vi "PulseTrain (G3)-Create (PWM).vi"(0 "State In":T1, 7 "Duty Cycle":dbl, 11 "error in (no error)":errorcluster) -> (4 "State Out":T1, 8 "Array":dbl[](array[numeric]), 15 "error out":errorcluster)   [LabVIEW 2015]
uses:
  Pulse Train-PWM State.ctl
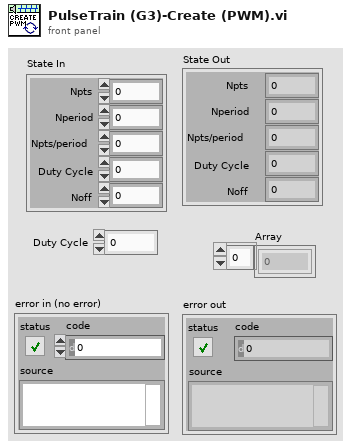
[diagram p1: front panel]
types:
  T1 = typedef "Pulse Train-PWM State.ctl" = cluster{"Npts":i32, "Nperiod":i32, "Npts/period":i32, "Duty Cycle":dbl, "Noff":i32}
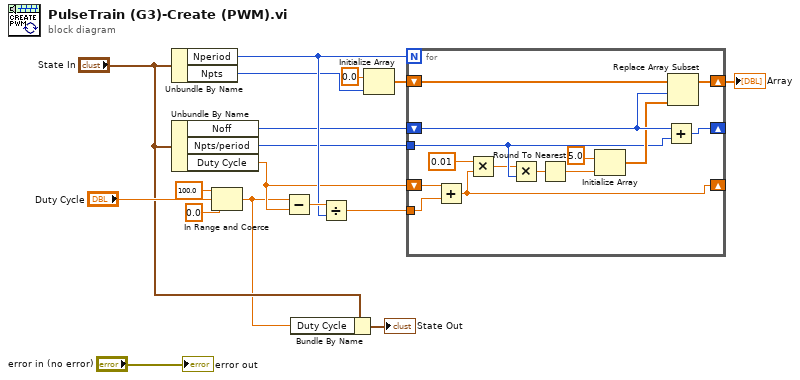
[diagram p0: block diagram]
diagram:
  n1 = Unbundle By Name("State In") -> ("Nperiod"=w13:i32, "Npts"=w7:i32)
  n2 = Unbundle By Name("State In") -> ("Noff"=w5:i32, "Npts/period"=w11:i32, "Duty Cycle"=w6:dbl)
  n3 = In Range and Coerce(upper limit=100.0, x="Duty Cycle", lower limit=0.0) -> (coerced(x)=w3:dbl)  [unwired: 1 out]
  n4 = Subtract(x=w3, y=w6) -> (x-y=w14:dbl)
  n5 = Bundle By Name(cluster="State In", "Duty Cycle"=w3) -> (→"State Out":T1)
  n6 = Divide(x=w14, y=w13) -> (x/y=w12:dbl)
  n7 = Initialize Array(0.0 ("element"), w7) -> (w16:dbl[])
  n8 = for {
    N: w13 -> [_]
    shift-right: [w26] -> w8
    shift-left: w16 -> [w27]
    shift-right: [w24] -> _
    shift-left: w5 -> [w25]
    tunnel: w12 -> [w30]
    tunnel: w11 -> [w21]
    shift-right: [w18] -> _
    shift-left: w6 -> [w31]
    n9 = Add(x=w31, y=w30) -> (x+y=w18:dbl)
    n10 = Multiply(x=0.01, y=w18) -> (x*y=w19:dbl)
    n11 = Multiply(x=w19, y=w21) -> (x*y=w28:dbl)
    n12 = Round To Nearest(number=w28) -> (nearest integer value=w20:dbl)
    n13 = Initialize Array(5.0, w20) -> (w22:dbl[])
    n14 = Add(x=w25, y=w21) -> (x+y=w24:i32)
    n15 = Replace Array Subset(array=w27, new element=w22, index=w25) -> (w26:dbl[])
  }
  "Array" <- w8
  "error out" <- "error in (no error)"
